vi "get_complete_dimension_names.vi"(8 "error in (no error)":errorcluster caption="错误输入（无错误）", 11 "MotorSystem输入":refnum<class "MotorSystem.lvclass">) -> (0 "error out":errorcluster caption="错误输出", 2 "dimension names":T1, 3 "MotorSystem输出":refnum<class "MotorSystem.lvclass">)   [LabVIEW 2016, in "MotionControl.lvlib" / "MotorSystem.lvclass"]
uses:
  <userlib>/MotionControl/MotorSystem/MotorSystem.lvclass
  <userlib>/MotionControl/MotorSystem/MotorSystem.lvclass/MotorSystem.ctl
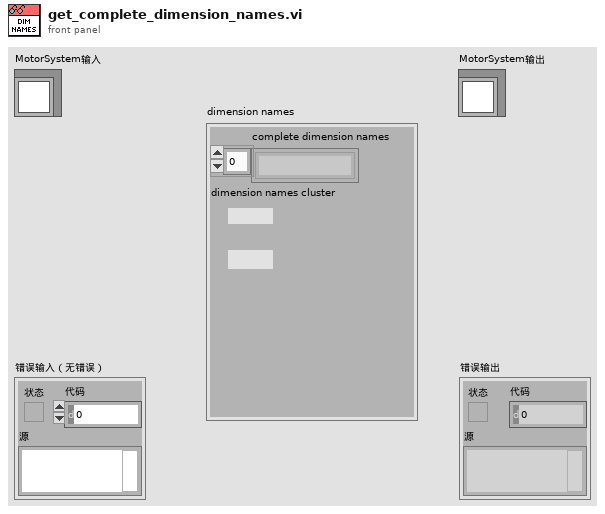
[diagram p1: front panel]
types:
  T1 = cluster{"complete dimension names":string[], "dimension names cluster ":cluster{"name 1":string, "name 2":string}}
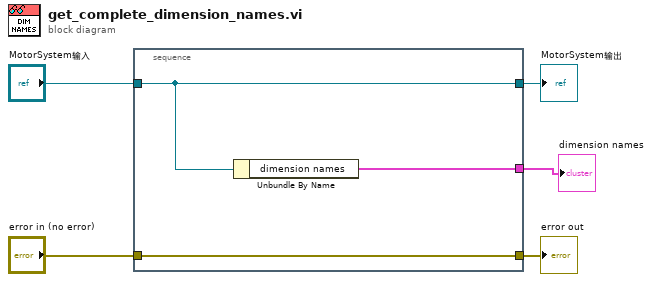
[diagram p0: block diagram]
diagram:
  n1 = stacked-sequence {
    tunnel: [w6] -> w5
    tunnel: [w8] -> w3
    tunnel: "MotorSystem输入" -> [w8]
    tunnel: [w7] -> w2
    tunnel: "error in (no error)" -> [w6]
    frame #0 {
      n2 = Unbundle By Name(w8) -> ("dimension names"=w7:T1)
    }
  }
  "error out" <- w5
  "MotorSystem输出" <- w3
  "dimension names" <- w2
